vi "Calibrate IMU Gyro.vi"(6 "Calib time (ms)":u32, 11 "I2CDevRef in":T1 {"Device Address" format="%.0x"}) -> (3 "I2CDevRef out":T1={"DevStatus"={"status"=FALSE, "code"=0, "source"=""}, "Controller"=enum."Controller 1", "Device Address"=0, "Handle"=0, "I2C Bus"=enum."Invalid"} {"Device Address" format="%.0x"})   [LabVIEW 2014]
uses:
  <vilib>/Rock Robotics/WPI/I2C/WPI_I2CDevRef.ctl
  <vilib>/Rock Robotics/SystemInterfaces/Typedef/FPGA_TypedefDigitalModule.ctl
  <vilib>/Rock Robotics/SystemInterfaces/i2clib/i2c_bus.ctl
  Robot Global Data.vi
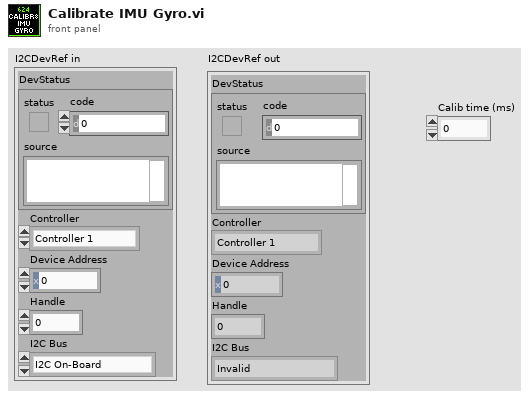
[diagram p1: front panel]
types:
  T1 = typedef "WPI_I2CDevRef.ctl" = cluster{"DevStatus":errorcluster, "Controller":T2, "Device Address":u8, "Handle":i32, "I2C Bus":T3}
  T2 = typedef "FPGA_TypedefDigitalModule.ctl" = enum16{"Controller 1"}
  T3 = typedef "i2c_bus.ctl" = enum16{"I2C On-Board", "I2C MXP", "Invalid"}
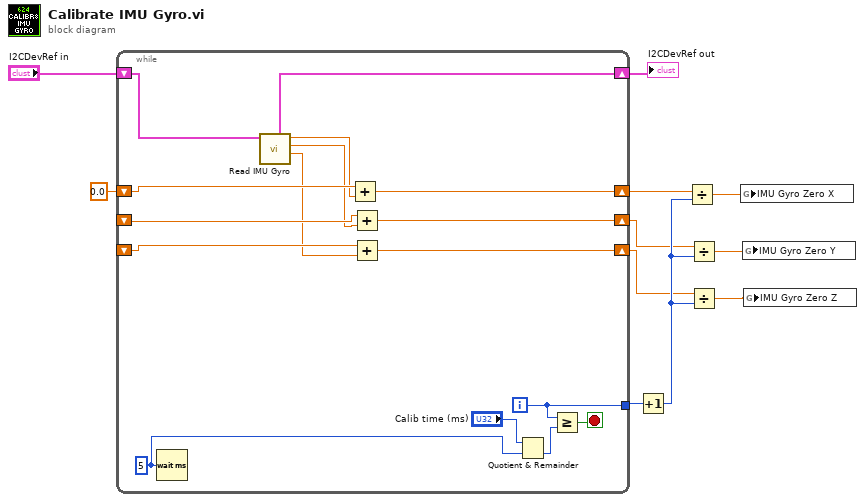
[diagram p0: block diagram]
diagram:
  n1 = while {
    shift-right: [w20] -> w10
    shift-left: "I2CDevRef in" -> [w21]
    tunnel: [w26] -> w8
    shift-right: [w19] -> w5
    shift-left: 0.0 -> [w22]
    shift-right: [w17] -> w4
    shift-left: _ -> [w18]
    shift-right: [w16] -> w3
    shift-left: _ -> [w15]
    i -> [w26]
    stop <- w27 stop-if-true
    w24 = u32 5 ("milliseconds to wait")
    n2 = Wait (ms)(milliseconds to wait=w24) -> ()  [unwired: 1 out]
    n3 = call "Read IMU Gyro.vi"("I2CDevRef"=w21) -> ("Z"=w12:dbl, "Y"=w13:dbl, "X"=w14:dbl, "I2CDevRef 2"=w20:T1)  [unwired: 7 in]
    n4 = Add(x=w22, y=w14) -> (x+y=w19:dbl)
    n5 = Add(x=w18, y=w13) -> (x+y=w17:dbl)
    n6 = Add(x=w15, y=w12) -> (x+y=w16:dbl)
    n7 = Quotient & Remainder(x="Calib time (ms)", y=w24) -> (floor(x/y)=w23:u32)  [unwired: 1 out]
    n8 = Greater Or Equal?(x=w26, y=w23) -> (x >= y?=w27:bool)
  }
  "I2CDevRef out" <- w10
  n9 = Increment(x=w8) -> (x+1=w6:i32)
  n10 = Divide(x=w5, y=w6) -> (x/y=w1:dbl)
  n11 = Divide(x=w4, y=w6) -> (x/y=w2:dbl)
  n12 = Divide(x=w3, y=w6) -> (x/y=w7:dbl)
  n13 = global write "Robot Global Data.vi" "IMU Gyro Zero X"(w1) -> ()
  n14 = global write "Robot Global Data.vi" "IMU Gyro Zero Y"(w2) -> ()
  n15 = global write "Robot Global Data.vi" "IMU Gyro Zero Z"(w7) -> ()
